vi "Get Category.vi"(8 "error in (no error)":errorcluster, 11 "SystemLink editor node in":refnum<class "SystemLink File editor node.lvclass">) -> (0 "error out":errorcluster, 2 "Category":string, 3 "SystemLink editor node out":refnum<class "SystemLink File editor node.lvclass">)   [LabVIEW 2015, in "SystemLink File editor node.lvclass"]
uses:
  SystemLink File editor node.lvclass
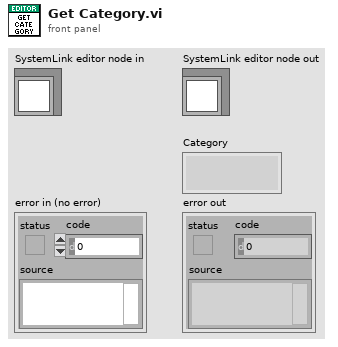
[diagram p1: front panel]
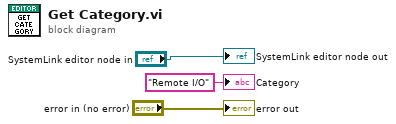
[diagram p0: block diagram]
diagram:
  "error out" <- "error in (no error)"
  "SystemLink editor node out" <- "SystemLink editor node in"
  "Category" <- "Remote I/O" ("Category")
